vi "Sample Transfer Check Containers.vi"(8 "error in (no error)":errorcluster, 11 "cRIO-CO2 in":refnum<class "cRIO-CO2.lvclass">) -> (0 "error out":errorcluster, 1 "Valid Containers?":bool, 3 "cRIO-CO2 out":refnum<class "cRIO-CO2.lvclass">, 4 "Message":string)   [LabVIEW 2015, in "cRIO-Carbondioxide.lvlib" / "cRIO-CO2.lvlib" / "cRIO-CO2.lvclass"]
uses:
  cRIO-CO2.lvclass
  cRIO-CO2.lvclass/cRIO-CO2.ctl
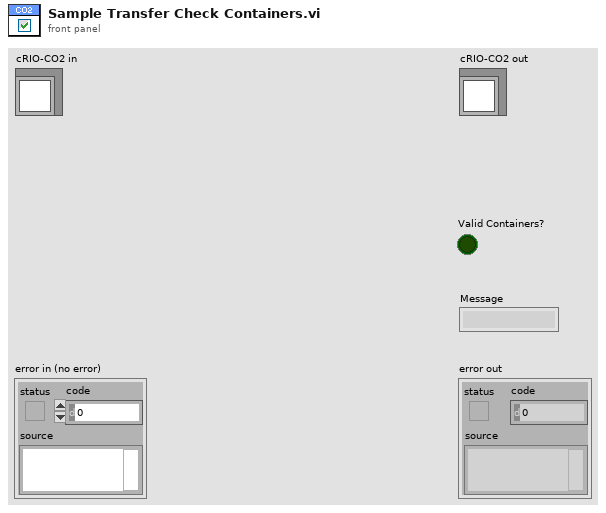
[diagram p1: front panel]
types:
  T1 = typedef "Sample Transfer Container Enumerator.ctl" = enum16{"None", "Sample 1", "Sample 2", "Sample 3", "Sample 4", "Sample 5", "Storage 01", "Storage 02", "Storage 03", "Storage 04", "Storage 05", "Storage 06", "Storage 07", "Storage 08", "Storage 09", "Storage 10", "Storage 11", "Storage 12", "Syringe", "Undefined"}
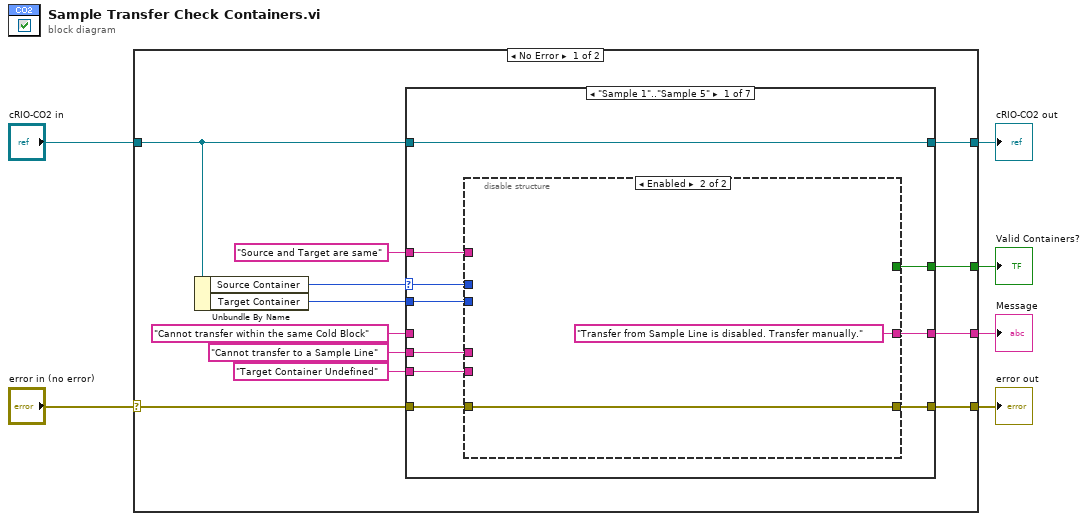
[diagram p0: block diagram]
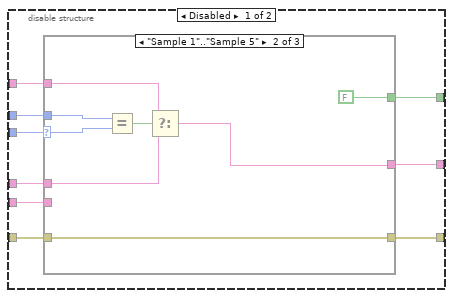
[diagram p2: hidden frame]
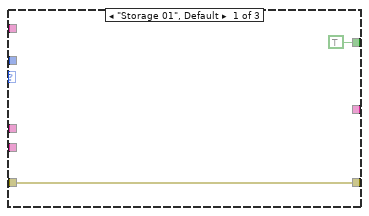
[diagram p3: hidden frame]
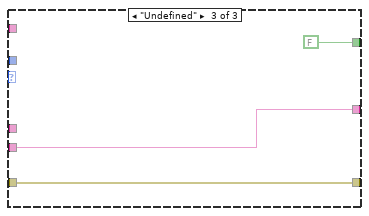
[diagram p4: hidden frame]
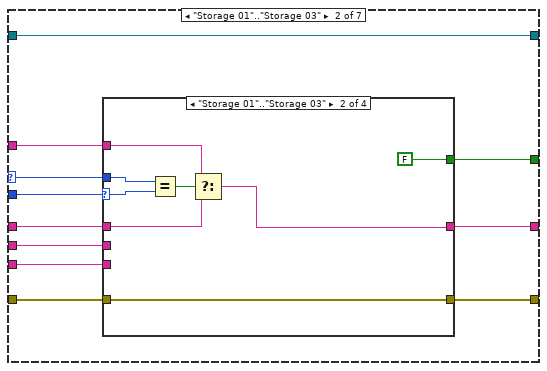
[diagram p5: hidden frame]
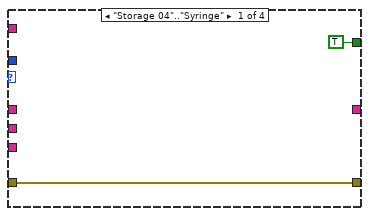
[diagram p6: hidden frame]
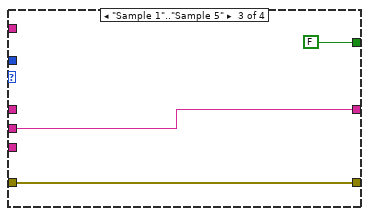
[diagram p7: hidden frame]
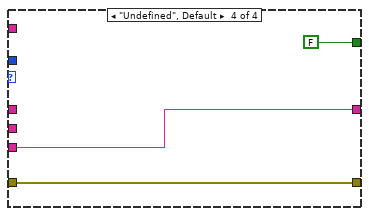
[diagram p8: hidden frame]
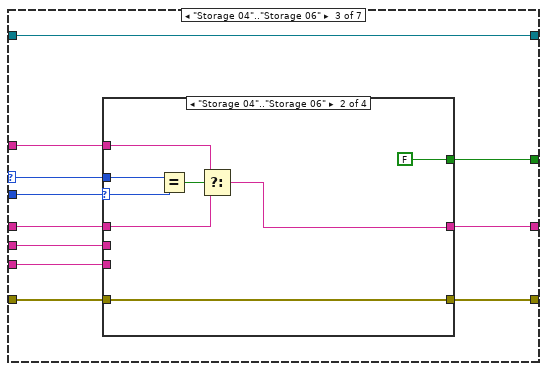
[diagram p9: hidden frame]
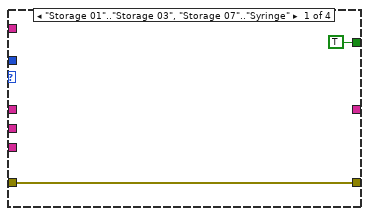
[diagram p10: hidden frame]
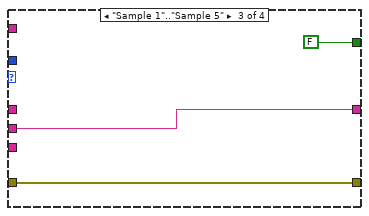
[diagram p11: hidden frame]
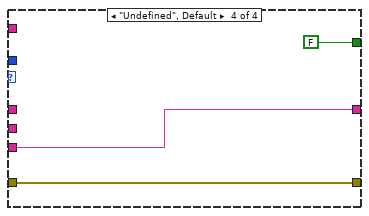
[diagram p12: hidden frame]
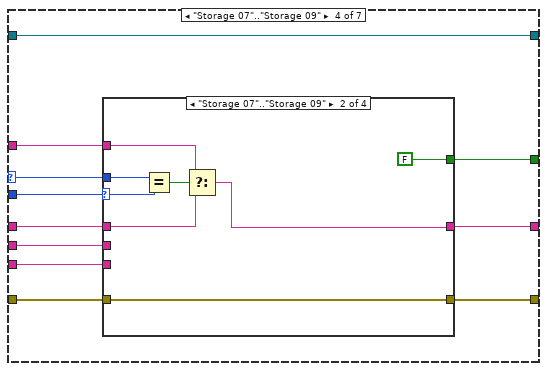
[diagram p13: hidden frame]
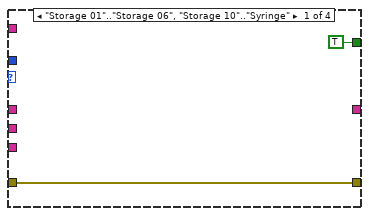
[diagram p14: hidden frame]
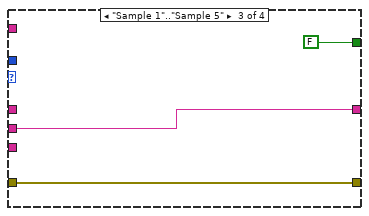
[diagram p15: hidden frame]
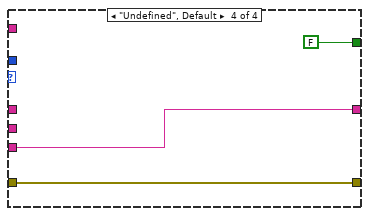
[diagram p16: hidden frame]
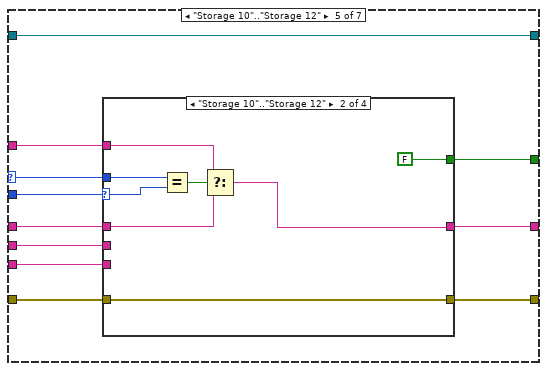
[diagram p17: hidden frame]
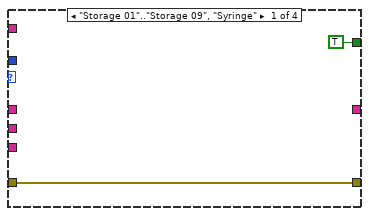
[diagram p18: hidden frame]
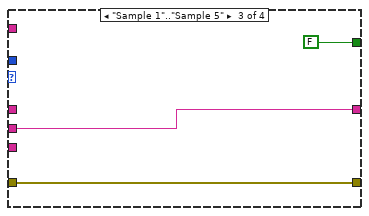
[diagram p19: hidden frame]
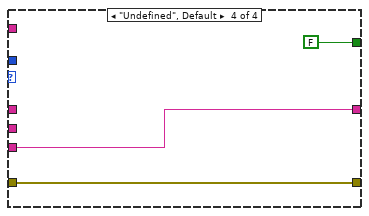
[diagram p20: hidden frame]
diagram:
  n1 = case shown="No Error" "error in (no error)" {
    selector: "error in (no error)" -> [w17 w187]
    tunnel: [w16 w187] -> w5
    tunnel: [w14 w186] -> w3
    tunnel: "cRIO-CO2 in" -> [w18 w186]
    tunnel: [w12 _] -> w2
    tunnel: [w11 _] -> w1
    frame No Error {
      n2 = Unbundle By Name(w18) -> ("Source Container"=w15:T1, "Target Container"=w13:T1)
      n3 = case shown="\"Sample 1\"..\"Sample 5\"" w15 {
        selector: w15 -> [w20 w54 w81 w108 w135 _ _]
        tunnel: w18 -> [w28 w63 w90 w117 w144 w170 w185]
        tunnel: w17 -> [w26 w61 w88 w115 w142 w168 w184]
        tunnel: [w25 w60 w87 w114 w141 w167 w184] -> w16
        tunnel: [w28 w63 w90 w117 w144 w170 w185] -> w14
        tunnel: w13 -> [w27 w62 w89 w116 w143 w169 _]
        tunnel: [w24 w59 w86 w113 w140 w166 FALSE] -> w12
        tunnel: [w23 w58 w85 w112 w139 w165 "Source Container Undefined"] -> w11
        tunnel: "Cannot transfer within the same Cold Block" -> [_ w57 w84 w111 w138 w164 _]
        tunnel: "Cannot transfer to a Sample Line" -> [w21 w56 w83 w110 w137 w163 _]
        tunnel: "Target Container Undefined" -> [w22 w55 w82 w109 w136 w162 _]
        tunnel: "Source and Target are same" -> [w19 w53 w80 w107 w134 w161 _]
        frame "Sample 1".."Sample 5" {
          n4 = disable-structure shown="Enabled" {
            disable-tunnel: w27 -> [w37 _]
            disable-tunnel: w26 -> [w36 w51]
            disable-tunnel: [w35 w51] -> w25
            disable-tunnel: [w34 _] -> w24
            disable-tunnel: [w33 "Transfer from Sample Line is disabled. Transfer manually."] -> w23
            disable-tunnel: w22 -> [w32 _]
            disable-tunnel: w21 -> [w31 _]
            disable-tunnel: w20 -> [w30 _]
            disable-tunnel: w19 -> [w29 _]
            frame Disabled {
              n5 = case shown="\"Sample 1\"..\"Sample 5\"" w37 {
                selector: w37 -> [_ w44 _]
                tunnel: w36 -> [w39 w46 w49]
                tunnel: [w39 w46 w49] -> w35
                tunnel: [TRUE FALSE FALSE] -> w34
                tunnel: [_ w41 w48] -> w33
                tunnel: w32 -> [_ _ w48]
                tunnel: w31 -> [_ w42 _]
                tunnel: w30 -> [_ w45 _]
                tunnel: w29 -> [_ w40 _]
                frame "Storage 01", Default {
                }
                frame "Sample 1".."Sample 5" {
                  n6 = Equal?(x=w45, y=w44) -> (x = y?=w43:bool)
                  n7 = Select(t=w40, s=w43, f=w42) -> (s? t:f=w41:string)
                }
                frame "Undefined" {
                }
              }
            }
            frame Enabled {
            }
          }
        }
        frame "Storage 01".."Storage 03" {
          n8 = case shown="\"Storage 01\"..\"Storage 03\"" w62 {
            selector: w62 -> [_ w69 _ _]
            tunnel: w61 -> [w65 w72 w75 w78]
            tunnel: [w65 w72 w75 w78] -> w60
            tunnel: [TRUE FALSE FALSE FALSE] -> w59
            tunnel: [_ w66 w74 w77] -> w58
            tunnel: w57 -> [_ w67 _ _]
            tunnel: w56 -> [_ _ w74 _]
            tunnel: w55 -> [_ _ _ w77]
            tunnel: w54 -> [_ w70 _ _]
            tunnel: w53 -> [_ w68 _ _]
            frame "Storage 04".."Syringe" {
            }
            frame "Storage 01".."Storage 03" {
              n9 = Equal?(x=w70, y=w69) -> (x = y?=w71:bool)
              n10 = Select(t=w68, s=w71, f=w67) -> (s? t:f=w66:string)
            }
            frame "Sample 1".."Sample 5" {
            }
            frame "Undefined", Default {
            }
          }
        }
        frame "Storage 04".."Storage 06" {
          n11 = case shown="\"Storage 04\"..\"Storage 06\"" w89 {
            selector: w89 -> [_ w96 _ _]
            tunnel: w88 -> [w92 w99 w102 w105]
            tunnel: [w92 w99 w102 w105] -> w87
            tunnel: [TRUE FALSE FALSE FALSE] -> w86
            tunnel: [_ w93 w101 w104] -> w85
            tunnel: w84 -> [_ w94 _ _]
            tunnel: w83 -> [_ _ w101 _]
            tunnel: w82 -> [_ _ _ w104]
            tunnel: w81 -> [_ w97 _ _]
            tunnel: w80 -> [_ w95 _ _]
            frame "Storage 01".."Storage 03", "Storage 07".."Syringe" {
            }
            frame "Storage 04".."Storage 06" {
              n12 = Equal?(x=w97, y=w96) -> (x = y?=w98:bool)
              n13 = Select(t=w95, s=w98, f=w94) -> (s? t:f=w93:string)
            }
            frame "Sample 1".."Sample 5" {
            }
            frame "Undefined", Default {
            }
          }
        }
        frame "Storage 07".."Storage 09" {
          n14 = case shown="\"Storage 07\"..\"Storage 09\"" w116 {
            selector: w116 -> [_ w123 _ _]
            tunnel: w115 -> [w119 w126 w129 w132]
            tunnel: [w119 w126 w129 w132] -> w114
            tunnel: [TRUE FALSE FALSE FALSE] -> w113
            tunnel: [_ w120 w128 w131] -> w112
            tunnel: w111 -> [_ w121 _ _]
            tunnel: w110 -> [_ _ w128 _]
            tunnel: w109 -> [_ _ _ w131]
            tunnel: w108 -> [_ w124 _ _]
            tunnel: w107 -> [_ w122 _ _]
            frame "Storage 01".."Storage 06", "Storage 10".."Syringe" {
            }
            frame "Storage 07".."Storage 09" {
              n15 = Equal?(x=w124, y=w123) -> (x = y?=w125:bool)
              n16 = Select(t=w122, s=w125, f=w121) -> (s? t:f=w120:string)
            }
            frame "Sample 1".."Sample 5" {
            }
            frame "Undefined", Default {
            }
          }
        }
        frame "Storage 10".."Storage 12" {
          n17 = case shown="\"Storage 10\"..\"Storage 12\"" w143 {
            selector: w143 -> [_ w150 _ _]
            tunnel: w142 -> [w146 w153 w156 w159]
            tunnel: [w146 w153 w156 w159] -> w141
            tunnel: [TRUE FALSE FALSE FALSE] -> w140
            tunnel: [_ w147 w155 w158] -> w139
            tunnel: w138 -> [_ w149 _ _]
            tunnel: w137 -> [_ _ w155 _]
            tunnel: w136 -> [_ _ _ w158]
            tunnel: w135 -> [_ w151 _ _]
            tunnel: w134 -> [_ w148 _ _]
            frame "Storage 01".."Storage 09", "Syringe" {
            }
            frame "Storage 10".."Storage 12" {
              n18 = Equal?(x=w151, y=w150) -> (x = y?=w152:bool)
              n19 = Select(t=w148, s=w152, f=w149) -> (s? t:f=w147:string)
            }
            frame "Sample 1".."Sample 5" {
            }
            frame "Undefined", Default {
            }
          }
        }
        frame "Syringe" {
          n20 = case shown="\"Sample 1\"..\"Sample 5\"" w169 {
            tunnel: w168 -> [w172 w174 w177 w180]
            tunnel: [w172 w174 w177 w180] -> w167
            tunnel: [TRUE FALSE FALSE FALSE] -> w166
            tunnel: [_ w173 w178 w179] -> w165
            tunnel: w164 -> [_ _ _ _]
            tunnel: w163 -> [_ w173 _ _]
            tunnel: w162 -> [_ _ _ w179]
            tunnel: w161 -> [_ _ w178 _]
            frame "Storage 01".."Storage 12" {
            }
            frame "Sample 1".."Sample 5" {
            }
            frame "Syringe" {
            }
            frame "Undefined", Default {
            }
          }
        }
        frame "Undefined", Default {
        }
      }
    }
    frame Error {
    }
  }
  "error out" <- w5
  "cRIO-CO2 out" <- w3
  "Valid Containers?" <- w2
  "Message" <- w1
